vi "Status Logger Unit Test VI.vi"() -> ()   [LabVIEW 2015]
uses:
  support/Status Logger/Status Log.ctl
panel:
  out "Staus Log Path":path
  in  "Status":string="Testowy status"
  out "error out":errorcluster
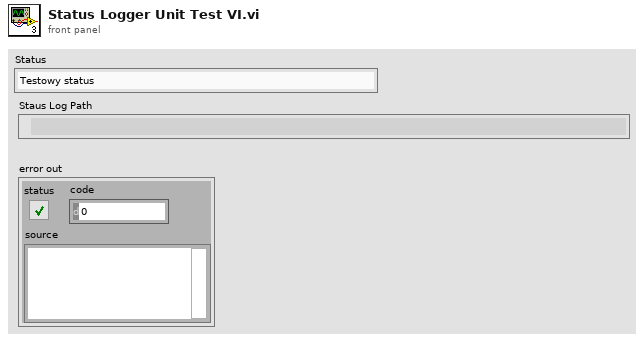
[diagram p1: front panel]
types:
  T1 = typedef "Status Log.ctl" = enum16{"Close file", "Open Status file", "Add Status", "Get file path"}
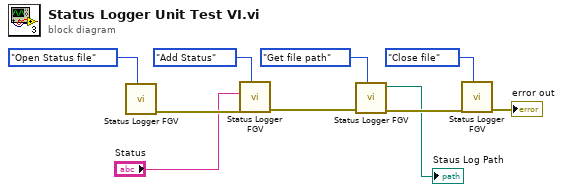
[diagram p0: block diagram]
diagram:
  n1 = call "Status Logger FGV.vi"("Action"=Status_Log."Open Status file") -> ("error out"=w9:errorcluster)  [unwired: 9 in, 1 out]
  n2 = call "Status Logger FGV.vi"("Action"=Status_Log."Add Status", "error in (no error)"=w9, "Status"="Status") -> ("error out"=w6:errorcluster)  [unwired: 7 in, 1 out]
  n3 = call "Status Logger FGV.vi"("Action"=Status_Log."Get file path", "error in (no error)"=w6) -> ("error out"=w4:errorcluster, "Staus Log Path"=→"Staus Log Path":path)  [unwired: 8 in]
  n4 = call "Status Logger FGV.vi"("Action"=Status_Log."Close file", "error in (no error)"=w4) -> ("error out"=→"error out":errorcluster)  [unwired: 8 in, 1 out]
